vi "Pre Launch Init.vi"(11 "IObserver in":refnum<class "IObserver.lvclass">) -> (0 "error out":errorcluster, 3 "IObserver out":refnum<class "IObserver.lvclass">)   [LabVIEW 2019, in "IObserver.lvlib" / "IObserver.lvclass"]
doc: "(<B>Filename</B>: Actor Framework.lvlib:Actor.lvclass:Pre Launch Init.vi)\n\nDefines behavior that occurs after the Launch Nested Actor method is invoked but before the actor's Actor Core method begins running.\n\nBy default, this method does nothing. A descendant class may override it to define behavior."
uses:
  <vilib>/gpm_packages/@cs/mva-core/Source/IObserver/IObserver/IObserver.lvclass
  C:/Program Files/National Instruments/LabVIEW 2019/vi.lib/ActorFramework/Actor/Actor.lvclass
  <vilib>/gpm_packages/@cs/event-logger/Source/Composed Log/Types/Log Level.ctl
  <vilib>/gpm_packages/@cs/mva-core/Source/IObserver/IObserver/IObserver.lvclass/IObserver.ctl
  <vilib>/gpm_packages/@cs/event-logger/Source/Composed Log/LoggerReference/LoggerReference.lvclass/LoggerReference.ctl
  <vilib>/ActorFramework/Actor/Actor.lvclass/Actor.ctl
  <vilib>/ActorFramework/Message Enqueuer/Message Enqueuer.lvclass/Message Enqueuer.ctl
  <vilib>/ActorFramework/Actor/Read Self Enqueuer.vi
  <vilib>/gpm_packages/@cs/event-logger/Source/Composed Log/LoggerReference/Log Event.vi
  <vilib>/ActorFramework/Message Enqueuer/Init from Existing Queue.vi
  <vilib>/gpm_packages/@cs/event-logger/Source/Composed Log/LoggerReference/Log.vi
  <vilib>/gpm_packages/@cs/event-logger/Source/Composed Log/LoggerReference/Get Valid Event Time.vi
  <vilib>/gpm_packages/@cs/event-logger/Source/Composed Log/LoggerReference/Remove Stale Logs.vi
  <vilib>/Utility/LVClass/Get LV Class Name.vi
  <vilib>/Utility/error.llb/Error Cluster From Error Code.vi
  <vilib>/ActorFramework/Message Enqueuer/Message Enqueuer.lvclass
  <vilib>/ActorFramework/Actor/Actor.lvclass
  <vilib>/gpm_packages/@cs/event-logger/Source/Composed Log/Composed Log.lvlib
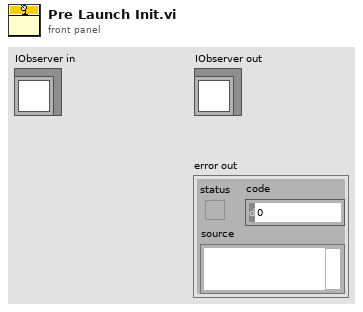
[diagram p1: front panel]
types:
  T1 = typedef "Composed Log.lvlib/Log Level.ctl" = enum16{"Debug", "Info", "Warning", "Error", "Critical"}
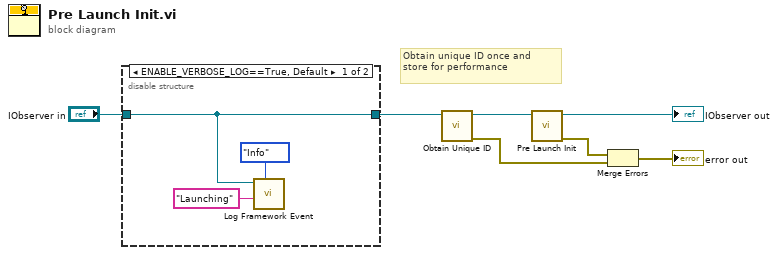
[diagram p0: block diagram]
diagram:
  # "Obtain unique ID once and\nstore for performance"
  n1 = disable-structure shown="ENABLE_VERBOSE_LOG==True, Default" {
    disable-tunnel: "IObserver in" -> [w8 w11]
    disable-tunnel: [w8 w11] -> w1
    frame condition #0 (active) {
      # "Log launch event by default"
      n2 = call <vilib>:"Log Framework Event.vi"("Event Level (Debug)"=Log_Level."Info", "Data To Log"="Launching", "IObserver in"=w8) -> ()  [unwired: 8 in, 1 out]
    }
    frame condition #1 {
      # "Remove all logging from this method"
    }
  }
  n3 = call <vilib>:"Obtain Unique ID.vi"("IObserver In"=w1) -> ("error out"=w2:errorcluster, "IObserver Out"=w4:refnum<class "IObserver.lvclass">)  [unwired: 9 in]
  n4 = call-parent "Pre Launch Init.vi"("Actor in"=w4) -> ("error out"=w7:errorcluster, "Actor out"=→"IObserver out":refnum<class "IObserver.lvclass">)  [unwired: 9 in]
  n5 = Merge Errors(w7, w2) -> (→"error out":errorcluster)
